vi "Dialog_Arrow Down on Listbox.vi"(11 "TreeControl in":refnum<vi>) -> (3 "discard":bool)   [LabVIEW 2023]
doc: "If one item is selected and it's the last item, and the down arrow is pressed, move to first item in listbox"
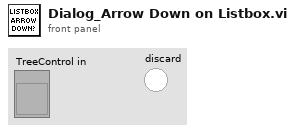
[diagram p1: front panel]
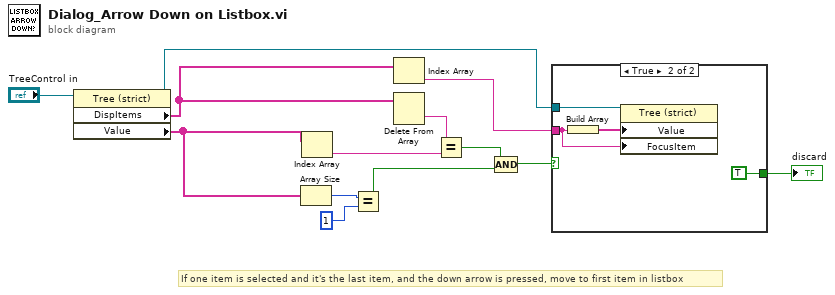
[diagram p0: block diagram]
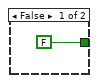
[diagram p2: hidden frame]
diagram:
  # "If one item is selected and it's the last item, and the down arrow is pressed, move to first item in listbox"
  n1 = property class="Tree (strict)"(reference="TreeControl in") -> (reference out=w13:refnum<vi>, "DispItems"=w12:string[], "Value"=w8:string[])  [unwired: 1 in, 1 out]
  n2 = Array Size(array=w8) -> (size(s)=w10:i32)
  n3 = Index Array(array=w8) -> (element=w4:string)  [unwired: 1 in]
  n4 = Equal?(x=w10, y=1) -> (x = y?=w7:bool)
  n5 = Index Array(array=w12) -> (element=w2:string)  [unwired: 1 in]
  n6 = Delete From Array(array=w12) -> (deleted portion=w3:string)  [unwired: 2 in, 1 out]
  n7 = Equal?(x=w3, y=w4) -> (x = y?=w1:bool)
  n8 = Compound Arithmetic op=AND(w1, w7) -> (w6:bool)
  n9 = case shown="True" w6 {
    tunnel: w13 -> [_ w18]
    tunnel: w2 -> [_ w15]
    tunnel: [FALSE ("discard") TRUE ("discard")] -> w5
    frame False {
    }
    frame True {
      n10 = Build Array(w15) -> (w17:string[])
      n11 = property class="Tree (strict)"(reference=w18, "Value"=w17, "FocusItem"=w15) -> ()  [unwired: 1 in, 2 out]
    }
  }
  "discard" <- w5
